vi "Find Item by Tag.vi"(9 "Tree Tag":string, 11 "All Data":refnum<class "Data Item.lvclass">[](array[class])) -> (1 "Index":i32, 2 "Data Item":refnum<class "Data Item.lvclass">, 3 "All Data out":refnum<class "Data Item.lvclass">[](array[class]))   [LabVIEW 2026, in "VILab.lvlib"]
uses:
  VILab.lvlib
  Classes/Data Item/Data Item.lvclass
panel:
  out "Found?":bool
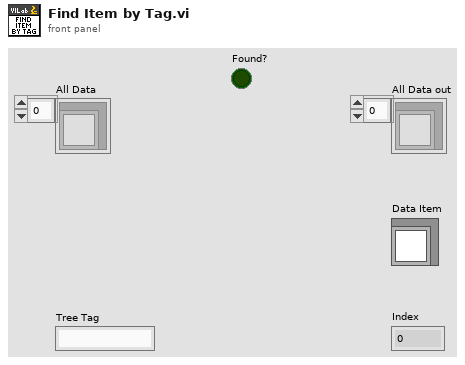
[diagram p1: front panel]
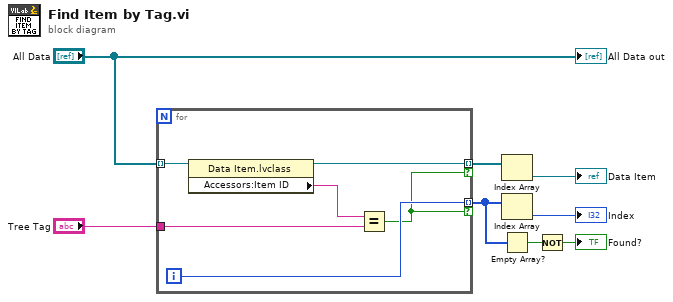
[diagram p0: block diagram]
diagram:
  n1 = for {
    tunnel: "All Data" -> [w14] mode=indexing
    tunnel: "Tree Tag" -> [w12]
    tunnel: [w11] -> w6 mode=indexing if=w9
    tunnel: [w10] -> w3 mode=indexing if=w9
    i -> [w10]
    n2 = property class="Data Item.lvclass"(reference=w14) -> (reference out=w11:refnum<class "Data Item.lvclass">, "Accessors:Item ID"=w13:string)  [unwired: 1 in, 1 out]
    n3 = Equal?(x=w13, y=w12) -> (x = y?=w9:bool)
  }
  n4 = Index Array(array=w6) -> (element=→"Data Item":refnum<class "Data Item.lvclass">)  [unwired: 1 in]
  n5 = Index Array(array=w3) -> (element=→"Index":i32)  [unwired: 1 in]
  n6 = Empty Array?(array=w3) -> (empty?=w2:bool)
  n7 = Not(x=w2) -> (.not. x?=→"Found?":bool)
  "All Data out" <- "All Data"
